vi "MReadParse.vi"(8 "error in (no error)":errorcluster, 11 "StrIn":string="M123mabcU3") -> (0 "error out":errorcluster, 1 "AllAck":bool, 2 "Modes":string[](array[string]), 3 "Values":dbl[](array[numeric]))   [LabVIEW 2016]
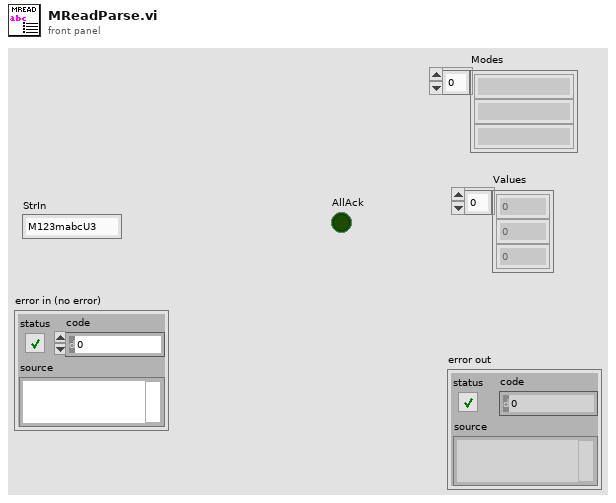
[diagram p1: front panel]
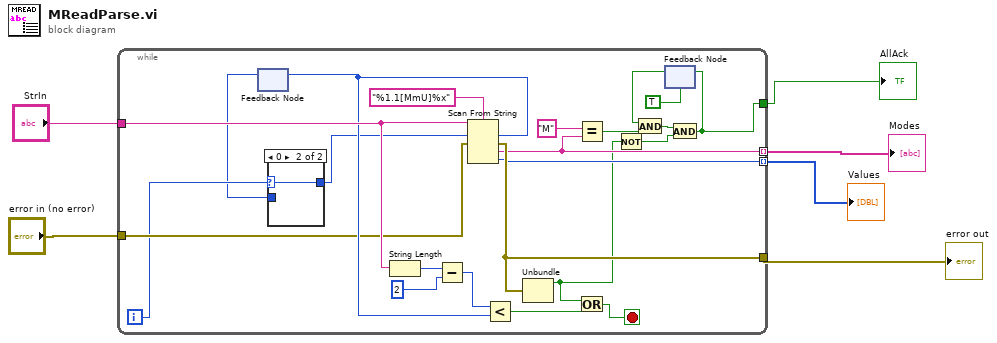
[diagram p0: block diagram]
diagram:
  n1 = while {
    tunnel: [w28] -> w5
    tunnel: "StrIn" -> [w24]
    tunnel: [w19] -> w4 mode=indexing
    tunnel: [w21] -> w3 mode=indexing
    tunnel: [w10] -> w2
    tunnel: "error in (no error)" -> [w14]
    i -> [w9]
    stop <- w22 stop-if-true
    n2 = feedback #1() -> (w7:u32)  [unwired: 1 in]
    n3 = case shown="0" w9 {
      selector: w9 -> [_ w31]
      tunnel: [w30 w31] -> w8
      tunnel: w7 -> [w30 _]
      frame Default {
      }
      frame 0 {
      }
    }
    n4 = String Length(string=w24) -> (length=w27:i32)
    n5 = Subtract(x=w27, y=2) -> (x-y=w25:i32)
    n6 = Scan From String(format string="%1.1[MmU]%x", input string=w24, initial scan location=w8, error in=w14) -> (offset past scan=w20:u32, error out=w28:errorcluster, output 1=w19:string, output 2=w21:u32)  [unwired: 2 in, 1 out]
    n7 = feedback-in #1(w20) -> ()
    n8 = Less?(x=w25, y=w20) -> (x < y?=w23:bool)
    n9 = Unbundle(w28) -> ("status"=w12:bool)  [unwired: 2 out]
    n10 = Equal?(x="M", y=w19) -> (x = y?=w17:bool)
    n11 = Or(x=w12, y=w23) -> (x .or. y?=w22:bool)
    n12 = Not(x=w12) -> (.not. x?=w13:bool)
    n13 = feedback #2(TRUE) -> (w15:bool)
    n14 = And(x=w15, y=w17) -> (x .and. y?=w11:bool)
    n15 = And(x=w11, y=w13) -> (x .and. y?=w10:bool)
    n16 = feedback-in #2(w10) -> ()
  }
  "Values" <- w3
  "Modes" <- w4
  "error out" <- w5
  "AllAck" <- w2
